vi "Define Events.vi"(8 "error in (no error)":errorcluster, 11 "Example Controller in":refnum<class "Example Controller.lvclass">) -> (0 "error out":errorcluster, 3 "Example Controller out":refnum<class "Example Controller.lvclass">)   [LabVIEW 2023, in "Example MVC Actors.lvlib" / "Example Controller.lvlib" / "Example Controller.lvclass"]
doc: "This dynamic dispatch VI has to be overriden by the concrete Souce Actor subclasses in order to define the event served by the source"
uses:
  Example Controller.lvclass
  Example Events/Double Array Event.lvclass
  Example Events/Timestamp Event.lvclass
  Example Events/Boolean Event.lvclass
  Example Controller Messages/Update Boolean Event Msg/Update Boolean Event Msg.lvclass
  Example Events/Inited At Event.lvclass
  Event/Event.lvclass/Event.ctl
  Event/Event.lvclass
  Controller/Controller.lvclass
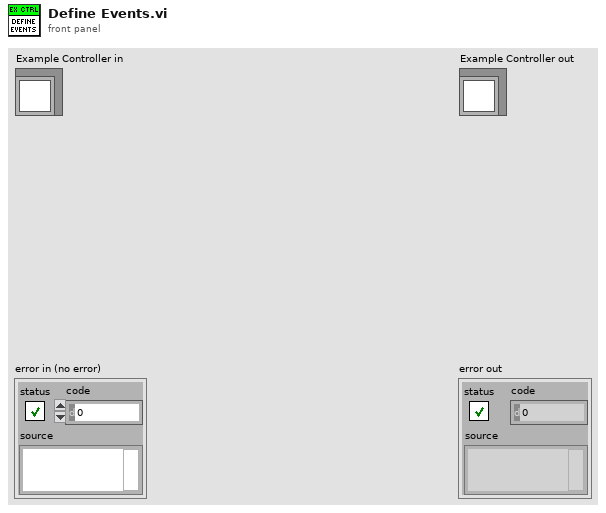
[diagram p1: front panel]
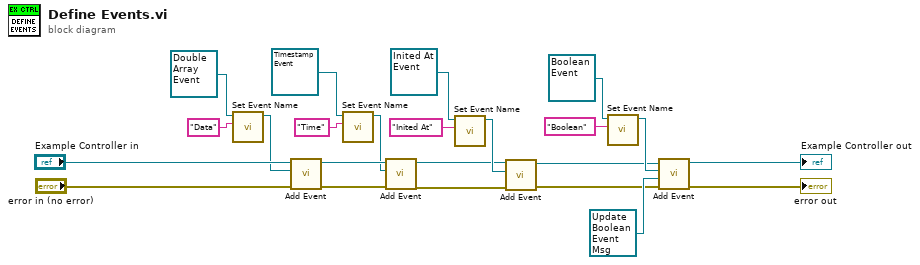
[diagram p0: block diagram]
diagram:
  n1 = call "Set Event Name.vi"("Name (Generic)"="Data", "Event In"=refnum<class "Double Array Event.lvclass"> refnum ("Double Array Event.lvclass")) -> ("Event Out"=w15:refnum<class "Double Array Event.lvclass">)  [unwired: 9 in]
  n2 = call "Add Event.vi"("error in (no error)"="error in (no error)", "Event"=w15, "Controller in"="Example Controller in") -> ("error out"=w11:errorcluster, "Controller out"=w16:refnum<class "Example Controller.lvclass">)  [unwired: 7 in]
  n3 = call "Set Event Name.vi"("Name (Generic)"="Time", "Event In"=refnum<class "Timestamp Event.lvclass"> refnum ("Timestamp Event.lvclass")) -> ("Event Out"=w14:refnum<class "Timestamp Event.lvclass">)  [unwired: 9 in]
  n4 = call "Add Event.vi"("error in (no error)"=w11, "Event"=w14, "Controller in"=w16) -> ("error out"=w4:errorcluster, "Controller out"=w5:refnum<class "Example Controller.lvclass">)  [unwired: 7 in]
  n5 = call "Set Event Name.vi"("Name (Generic)"="Inited At", "Event In"=refnum<class "Inited At Event.lvclass"> refnum ("Inited At Event.lvclass")) -> ("Event Out"=w6:refnum<class "Inited At Event.lvclass">)  [unwired: 9 in]
  n6 = call "Add Event.vi"("error in (no error)"=w4, "Event"=w6, "Controller in"=w5) -> ("error out"=w2:errorcluster, "Controller out"=w3:refnum<class "Example Controller.lvclass">)  [unwired: 7 in]
  n7 = call "Set Event Name.vi"("Name (Generic)"="Boolean", "Event In"=refnum<class "Boolean Event.lvclass"> refnum ("Example Source.lvlib:Boolean Event.lvclass")) -> ("Event Out"=w13:refnum<class "Boolean Event.lvclass">)  [unwired: 9 in]
  n8 = call "Add Event.vi"("error in (no error)"=w2, "Controller Event Handler"=refnum<class "Update Boolean Event Msg.lvclass"> refnum ("Example Source.lvlib:Update Boolean Msg.lvclass"), "Event"=w13, "Controller in"=w3) -> ("error out"=→"error out":errorcluster, "Controller out"=→"Example Controller out":refnum<class "Example Controller.lvclass">)  [unwired: 6 in]
